vi "Controller - State Exit.vi"(8 "error in (no error)":errorcluster, 11 "View Model":T1) -> (0 "error out":errorcluster, 3 "View Model":T1)   [LabVIEW 2017]
doc: "Provide processing of exit current state of Car Wash controller"
uses:
  View Model/Controls/View Model.ctl
  Configuration Database/Controls/Config Model.ctl
  Configuration Database/Controls/Config Commands.ctl
  Configuration Database/Controls/Congif Data.ctl
  View Model/Controls/Shared Model.ctl
  Error Handler/Controls/Error Model.ctl
  Error Handler/Controls/Error Data.ctl
  Error Handler/Controls/Error Type.ctl
  Controls/Car Wash Model.ctl
  Controls/Controller Overhead.ctl
  Controls/Vehicle Location.ctl
  Controls/Car Wash States.ctl
  Controls/CarWash CMD.ctl
  Views/Wash Display Console View/Controls/Car Wash Indicators.ctl
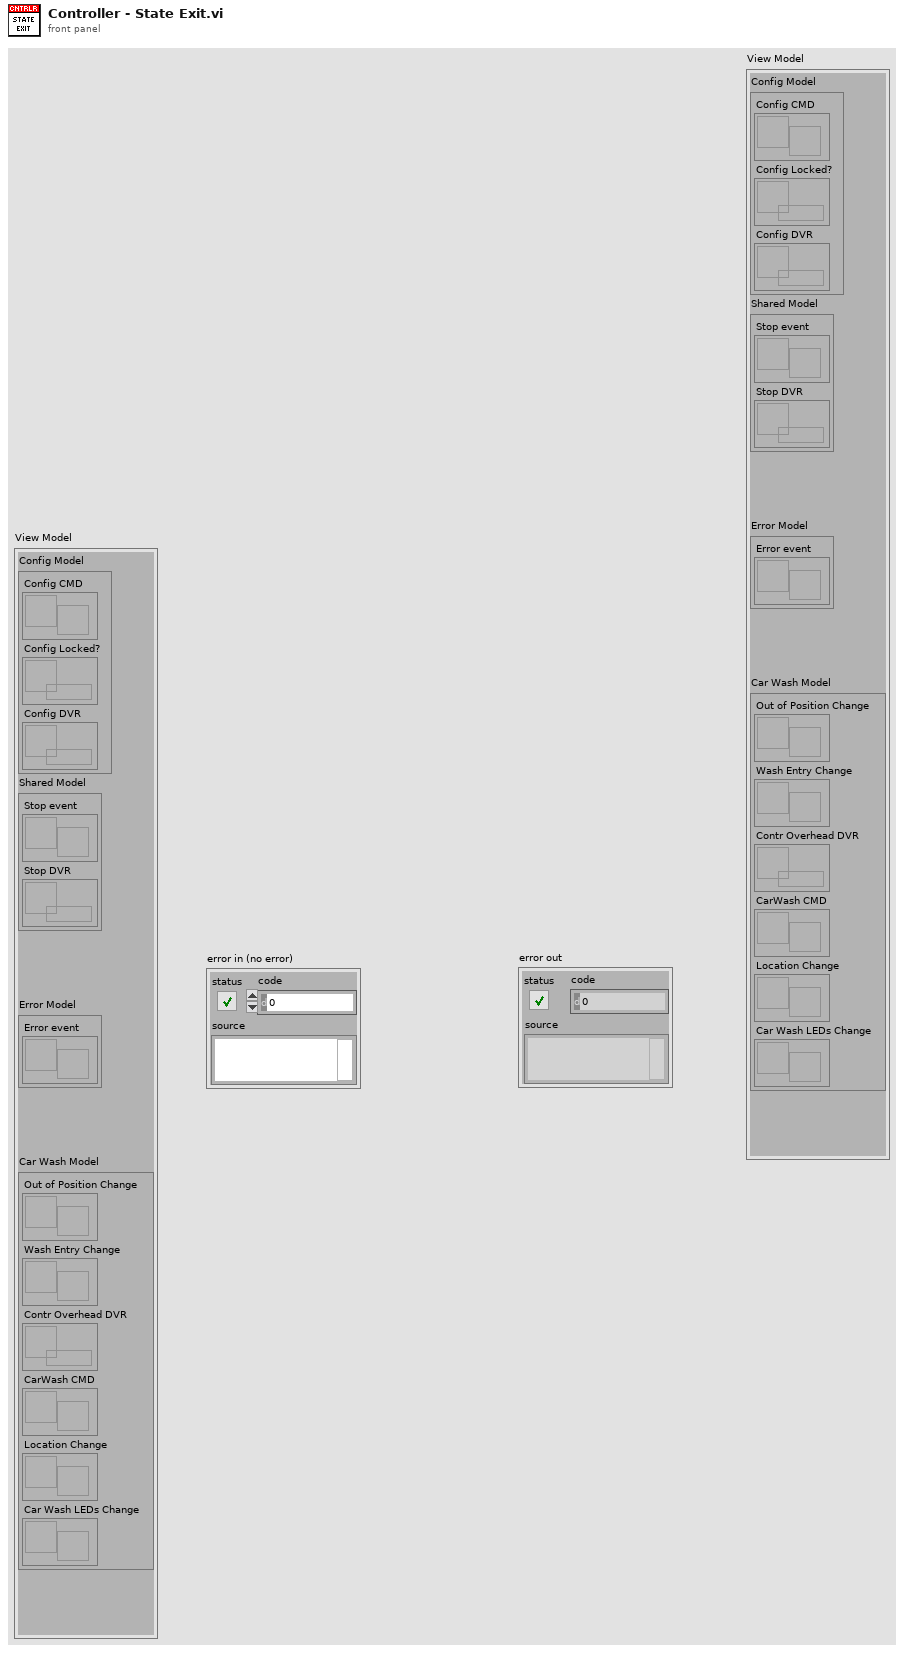
[diagram p1: front panel]
types:
  T1 = typedef "View Model.ctl" = cluster{"Config Model":T2, "Shared Model":T3, "Error Model":T4, "Car Wash Model":T5}
  T2 = typedef "Config Model.ctl" = cluster{"Config CMD":refnum<user-event>, "Config Locked?":refnum<data-value>, "Config DVR":refnum<data-value>}
  T3 = typedef "Shared Model.ctl" = cluster{"Stop event":refnum<user-event>, "Stop DVR":refnum<data-value>}
  T4 = typedef "Error Model.ctl" = cluster{"Error event":refnum<user-event>}
  T5 = typedef "Car Wash Model.ctl" = cluster{"Out of Position Change":refnum<user-event>, "Wash Entry Change":refnum<user-event>, "Contr Overhead DVR":refnum<data-value>, "CarWash CMD":refnum<user-event>, "Location Change":refnum<user-event>, "Car Wash LEDs Change":refnum<user-event>}
  T6 = typedef "Car Wash States.ctl" = enum16{"Initial", "Wait for start", "Start", "Wait for vehicle", "Wash Step Execution", "Wash Step/Cycle Complete", "Wash Exit", "Wash Abort/Terminate"}
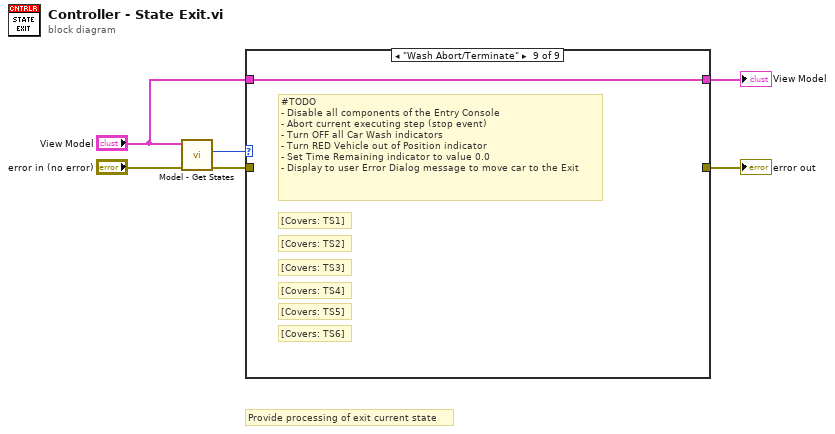
[diagram p0: block diagram]
diagram:
  # "Provide processing of exit current state"
  n1 = call "Model - Get States.vi"("error in (no error)"="error in (no error)", "View Model"="View Model") -> ("error out"=w3:errorcluster, "CarWash State"=w4:T6)  [unwired: 6 in, 2 out]
  n2 = case shown="\"Wash Abort/Terminate\"" w4 {
    tunnel: "View Model" -> [w8 w9 w10 w11 w12 w13 w14 w15 w16]
    tunnel: [w8 w9 w10 w11 w12 w13 w14 w15 w16] -> w1
    tunnel: w3 -> [w7 _ _ _ _ _ _ _ _]
    tunnel: [w7 _ _ _ _ _ _ _ _] -> w2
    frame Default {
    }
    frame "Initial" {
    }
    frame "Wait for start" {
    }
    frame "Start" {
    }
    frame "Wait for vehicle" {
    }
    frame "Wash Step Execution" {
    }
    frame "Wash Step/Cycle Complete" {
      # "[Covers: WC3C]"
      # "[Covers: WC3B]"
      # "[Covers: WC3A]"
      # "[Covers: WC2C]"
      # "[Covers: WC2B]"
      # "[Covers: WC2A]"
      # "[Covers: WC3]"
      # "[Covers: WC2]"
      # "#TODO\nTurn RED Vehicle out of Position indicator;\nIf the completed wash step was last\nthen -Turn OFF all Car wash indicators\n  - Wait until user move car position to Exit\nelse\n  - Turn on next Car Wash indicator corresponding\n     to next wash step\n  - Wait until user move car to the appropriate station"
    }
    frame "Wash Exit" {
      # "[Covers: WE4]"
      # "[Covers: WE3]"
      # "[Covers: WE2]"
      # "[Covers: WE1]"
      # "#TODO\n-Turn OFF all Car wash indicators\n- Wait until user move car position to Exit AND\n   reposition vehicle to the Entry position\n- Transition to Initial state"
    }
    frame "Wash Abort/Terminate" {
      # "[Covers: TS6]"
      # "[Covers: TS5]"
      # "[Covers: TS4]"
      # "[Covers: TS3]"
      # "[Covers: TS2]"
      # "[Covers: TS1]"
      # "#TODO\n- Disable all components of the Entry Console\n- Abort current executing step (stop event)\n- Turn OFF all Car Wash indicators\n- Turn RED Vehicle out of Position indicator\n- Set Time Remaining indicator to value 0.0\n- Display to user Error Dialog message to move car to the Exit"
    }
  }
  "error out" <- w2
  "View Model" <- w1
